vi "Scan.vi"(1 "Y Samples":u16=100 min=1 step=1, 2 "Y End  (um)":dbl=100.0 min=0.0 max=100.0 step=0.2 format="%.3f", 3 "Y Start  (um)":dbl min=0.0 max=100.0 step=0.5 format="%.3f", 7 "X Samples":u16=100 min=1 step=1, 8 "X End  (um)":dbl=100.0 min=0.0 max=100.0 step=0.2 format="%.3f", 9 "X Start  (um)":dbl min=0.0 max=100.0 step=0.5 format="%.3f") -> (0 "Y":dbl, 4 "XY Graph":cluster{"X":dbl[], "Y":dbl[]}[](graph), 6 "X":dbl)   [LabVIEW 2013]
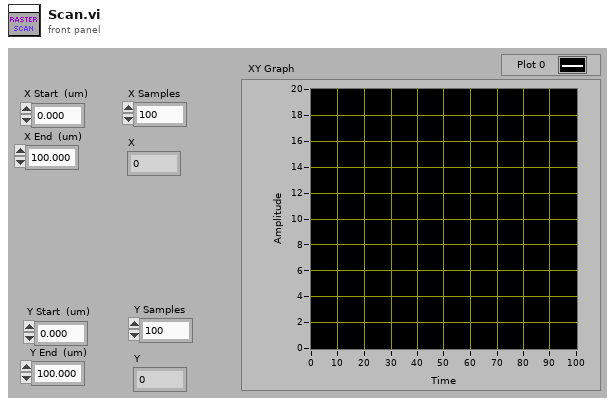
[diagram p1: front panel]
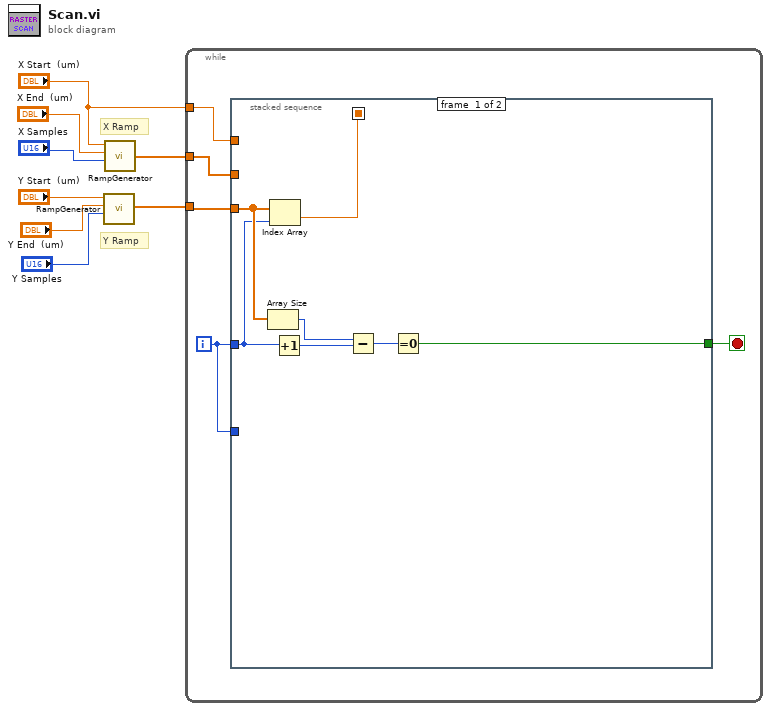
[diagram p0: block diagram]
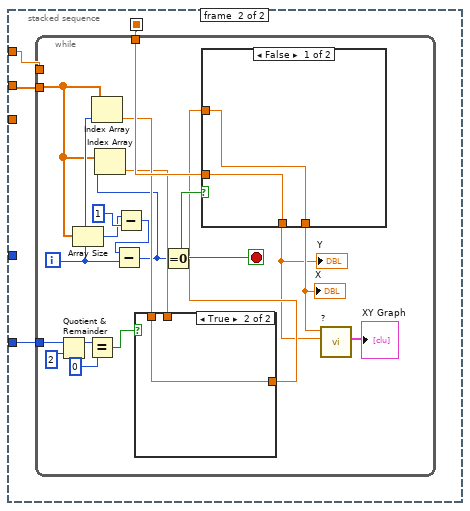
[diagram p2: hidden frame]
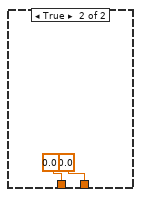
[diagram p4: hidden frame]
diagram:
  # "X Ramp"
  # "Y Ramp"
  n1 = call <instrlib>:"RampGenerator.vi"("Number of Positions"="Y Samples", "End  (um)"="Y End  (um)", "Start  (um)"="Y Start  (um)") -> ("Array"=w2:dbl[])  [unwired: 1 in]
  n2 = call <instrlib>:"RampGenerator.vi"("Number of Positions"="X Samples", "End  (um)"="X End  (um)", "Start  (um)"="X Start  (um)") -> ("Array"=w8:dbl[])  [unwired: 1 in]
  n3 = while {
    tunnel: w8 -> [w12]
    tunnel: w2 -> [w13]
    tunnel: "X Start  (um)" -> [w10]
    i -> [w9]
    stop <- w11 stop-if-true
    # "X Ramp Generator"
    n4 = stacked-sequence {
      seq-local: [w14 _] -> [_ w22]
      tunnel: w13 -> [w20 _]
      tunnel: [w18 _] -> w11
      tunnel: w9 -> [w16 _]
      tunnel: w12 -> [_ w24]
      tunnel: w10 -> [_ w23]
      tunnel: w9 -> [_ w21]
      frame #0 {
        n5 = Array Size(array=w20) -> (size(s)=w17:i32)
        n6 = Index Array(array=w20, index=w16) -> (element=w14:dbl)
        n7 = Increment(x=w16) -> (x+1=w15:i32)
        n8 = Subtract(x=w17, y=w15) -> (x-y=w19:i32)
        n9 = Equal To 0?(x=w19) -> (x = 0?=w18:bool)
      }
      frame #1 {
        n10 = while {
          tunnel: w24 -> [w33]
          tunnel: w23 -> [_]
          tunnel: w22 -> [w41]
          tunnel: w21 -> [w40]
          i -> [w42]
          stop <- w43 stop-if-true
          n11 = Quotient & Remainder(x=w40, y=2) -> (x-y*floor(x/y)=w38:i32)  [unwired: 1 out]
          n12 = Array Size(array=w33) -> (size(s)=w27:i32)
          n13 = Equal?(x=w38, y=0) -> (x = y?=w37:bool)
          n14 = Index Array(array=w33, index=w42) -> (element=w35:dbl)
          n15 = Subtract(x=w27, y=1) -> (x-y=w26:i32)
          n16 = Subtract(x=w26, y=w42) -> (x-y=w25:i32)
          n17 = Index Array(array=w33, index=w25) -> (element=w32:dbl)
          n18 = case shown="True" w37 {
            tunnel: w35 -> [_ w45]
            tunnel: [w44 w45] -> w34
            tunnel: w32 -> [w44 _]
            frame False {
            }
            frame True {
            }
          }
          n19 = Equal To 0?(x=w25) -> (x = 0?=w43:bool)
          n20 = case shown="False" w43 {
            tunnel: w34 -> [w46 _]
            tunnel: w41 -> [w47 _]
            tunnel: [w46 0.0 ("Numeric")] -> w29
            tunnel: [w47 0.0 ("Numeric")] -> w28
            frame False {
            }
            frame True {
              # "X AXIS SCAN"
            }
          }
          "X" <- w29
          "Y" <- w28
          n21 = call "?"("Y Input"=w28, "X Input"=w29) -> ("XY Graph"=→"XY Graph":cluster{"X":dbl[], "Y":dbl[]}[])  [unwired: 8 in, 1 out]
        }
      }
    }
  }
